vi "generar_frec.vi"(8 "error in (no error)":errorcluster, 10 "Data":variant) -> (0 "error out":errorcluster, 3 "Prueba04 out":refnum<class "Prueba04.lvclass">)   [LabVIEW 2019, in "Prueba04.lvclass"]
uses:
  Prueba04.lvclass
  Prueba/Queues/Private Controls/Control HMI Data Cluster.ctl
  Prueba/Queues/Private Controls/Estados.ctl
panel:
  out "error out 2":errorcluster
  in  "error in":errorcluster
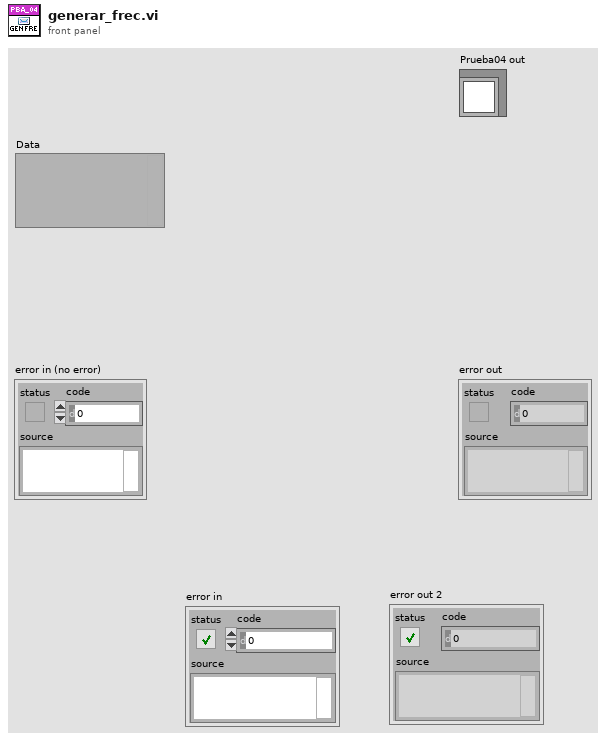
[diagram p1: front panel]
types:
  T1 = typedef "Control HMI Data Cluster.ctl" = cluster{"Estados":T2, "Data":variant}
  T2 = typedef "Estados.ctl" = enum16{"CargaReferencias", "LeerArchivoConfiguracion", "RevisaTipoGenerador", "inicio", "conf_instru", "escribe_frec", "lee_BD", "lee_referencia", "guardarVrefA", "guardarVrefC", "guardarVrefZ", "FrecAmp_A1", "FrecAmp_C1", "FrecAmp_Z1", "FrecAmp_A2", "FrecAmp_C2", "FrecAmp_Z2", "iniciarGEN", "monitoreo", "detenerGEN", "crea_voltajes_prueba_A", "crea_voltajes_prueba_C", "crea_voltajes_prueba_Z", "voltajeInicialA2", "voltajeInicialC2", "voltajeInicialZ2", "actualizarVrefA", "actualizarVrefC", "actualizarVrefZ", "ingresaMedicionesA", "ingresaMedicionesC", "ingresaMedicionesZ", "cumplimiento", "listo_evaluar", "evaluar", "final", "guardaMedicionesA", "guardaMedicionesC", "guardaMedicionesZ", "ultimaFrec", "generaA2", "detieneA2", "salir", "Error"}
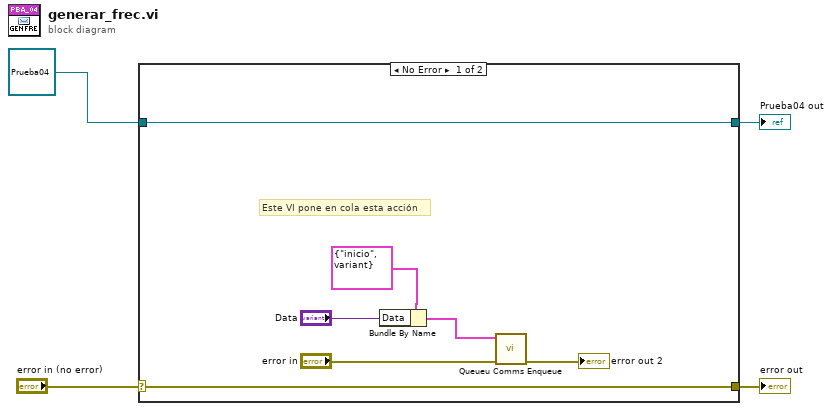
[diagram p0: block diagram]
diagram:
  n1 = case shown="No Error" "error in (no error)" {
    selector: "error in (no error)" -> [w10 w13]
    tunnel: [w10 w13] -> w3
    tunnel: [w11 w12] -> w1
    tunnel: refnum<class "Prueba04.lvclass"> refnum ("Prueba04 in") -> [w11 w12]
    frame No Error {
      # "Este VI pone en cola esta acción"
      n2 = Bundle By Name(cluster=T1 {"Estados"=enum."inicio", "Data"=variant} ("Module Dat Cluster"), "Data"="Data") -> (w5:T1)
      n3 = call "Queueu Comms Enqueue.vi"("error in"="error in", "Element"=w5) -> ("error out"=→"error out 2":errorcluster)  [unwired: 8 in, 1 out]
    }
    frame Error {
    }
  }
  "error out" <- w3
  "Prueba04 out" <- w1
